vi "Connect.vi"(8 "error in (no error)":errorcluster caption="entrée d'erreur (pas d'erreur)", 11 "Database Drivers en entrée":refnum<class "Database Drivers.lvclass">) -> (0 "error out":errorcluster caption="sortie d'erreur", 3 "Database Drivers en sortie":refnum<class "Database Drivers.lvclass">)   [LabVIEW 2020, in "Library Instrument & Equipement.lvlib" / "Library Database.lvlib" / "Database Drivers.lvclass"]
uses:
  Database Drivers.lvclass
  <vilib>/addons/database/Connection.llb/DB Tools Open Connec (String).vi
  Database Drivers.lvclass/Database Drivers.ctl
  <vilib>/addons/database/NI_Database_API.lvlib
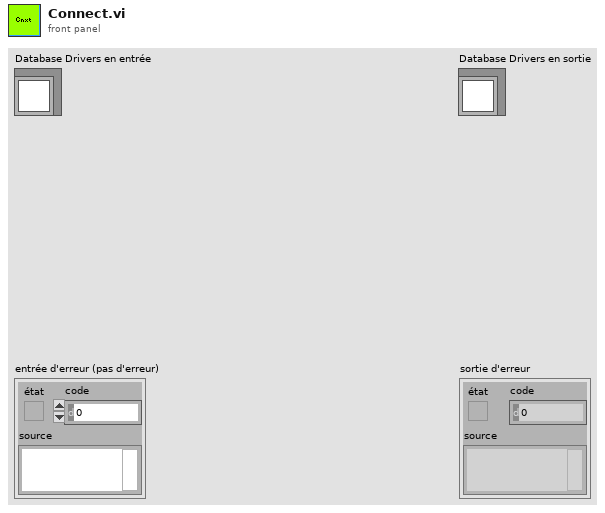
[diagram p1: front panel]
types:
  T1 = typedef "NI_Database_API.lvlib/Conn ObjectReference.ctl" = refnum<k1>
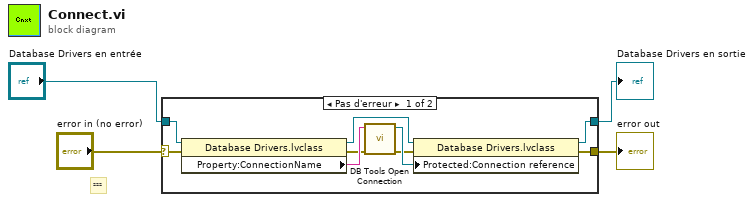
[diagram p0: block diagram]
diagram:
  # "²²²"
  n1 = case shown="Pas d'erreur" "error in (no error)" {
    selector: "error in (no error)" -> [w8 w15]
    tunnel: [w5 w15] -> w3
    tunnel: [w13 w14] -> w1
    tunnel: "Database Drivers en entrée" -> [w12 w14]
    frame No Error {
      n2 = property class="Database Drivers.lvclass"(reference=w12, error in=w8) -> (reference out=w11:refnum<class "Database Drivers.lvclass">, error out=w7:errorcluster, "Property:ConnectionName"=w10:string)
      n3 = call-poly <vilib>:"DB Tools Open Connection.vi"("error in (no error)"=w7, "connection information"=w10) -> ("error out"=w6:errorcluster, "connection reference"=w9:T1)  [unwired: 6 in]
      n4 = property class="Database Drivers.lvclass"(reference=w11, error in=w6, "Protected:Connection reference"=w9) -> (reference out=w13:refnum<class "Database Drivers.lvclass">, error out=w5:errorcluster)
    }
    frame Error {
    }
  }
  "error out" <- w3
  "Database Drivers en sortie" <- w1
